vi "Global Tektronix Report Cells.vi"() -> ()   [LabVIEW 2019]
panel:
  in  "AFG Opt Cell":string="Q5"
  in  "DVM Opt Cell":string="Q4"
  in  "Bandwidth Cell":string="Q3"
  in  "Channel Num Cell":string="Q2"
  in  "Model Cell 2":string="G1"
  in  "L. Results Col index":dbl=7.0
  in  "As Left Col index":dbl=6.0
  in  "F. Results Col index":dbl=5.0
  in  "As Found Col index":dbl=4.0
  in  "Nominal Col index":dbl=3.0
  in  "Funtion Col index":dbl=2.0
  in  "Local Path":path
  in  "Path":path=path "\\\\global.tektronix.net\\global/namerica/service/Completed Datasheets/Automation Completed"
  in  "File Name":string="\\\\global.tektronix.net\\global\\namerica\\service\\Completed Datasheets\\Automation Completed\\"
  in  "Proc Cell":string="M10"
  in  "FW Rev Cell":string="M9"
  in  "Max Col":string="I"
  in  "Uncert Col":string="K"
  in  "Units Col":string="J"
  in  "Nominal Col":string="C"
  in  "Function Col":string="B"
  in  "Min Col":string="H"
  in  "L. Result Col":string="G"
  in  "F. Result Col":string="E"
  in  "As Left Col":string="F"
  in  "As Found Col":string="D"
  in  "First Data Cell":string="D14"
  in  "ID Number Cell":string="C9"
  in  "Cal Date Cell":string="H9"
  in  "MFR Cell":string="C8"
  in  "Model Cell":string="H8"
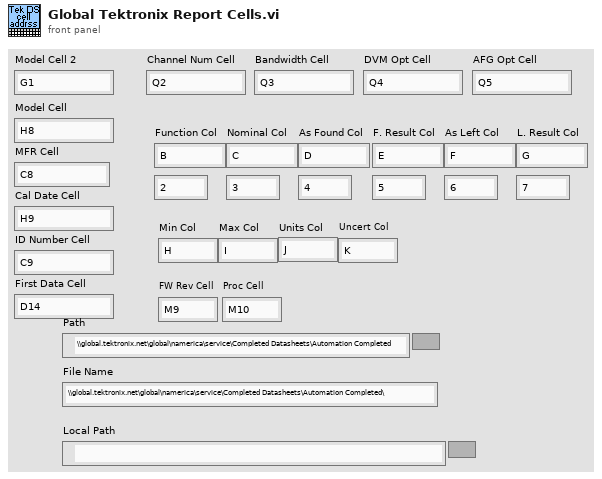
[diagram p1: front panel]
diagram:
